vi "ReadStringData.vi"(8 "Error In":errorcluster caption="エラー入力", 10 "データ":T2, 11 "refnum":T1) -> (0 "Error Out":errorcluster caption="エラー出力", 2 "文字列":string, 3 "refnum out":T1 caption="refnum出力")   [LabVIEW 2014]
doc: "iniファイルから文字列データを読み込みます。"
uses:
  <vilib>/Utility/config.llb/NI_LVConfig.lvlib
  <vilib>/Utility/config.llb/Write Key (String).vi
  <vilib>/Utility/config.llb/Read Key (String).vi
  <vilib>/Utility/config.llb/Config Data RefNum.ctl
panel:
  # "■Iniファイルから文字列データを読込む"
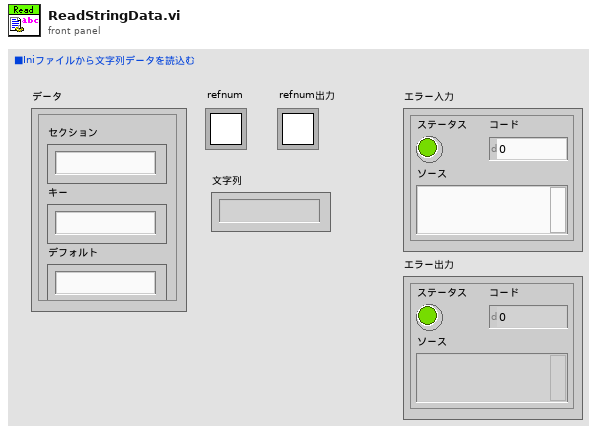
[diagram p1: front panel]
types:
  T1 = typedef "NI_LVConfig.lvlib/Config Data RefNum.ctl" = refnum<k1>
  T2 = cluster{"セクション":string, "キー":string, "デフォルト":string}
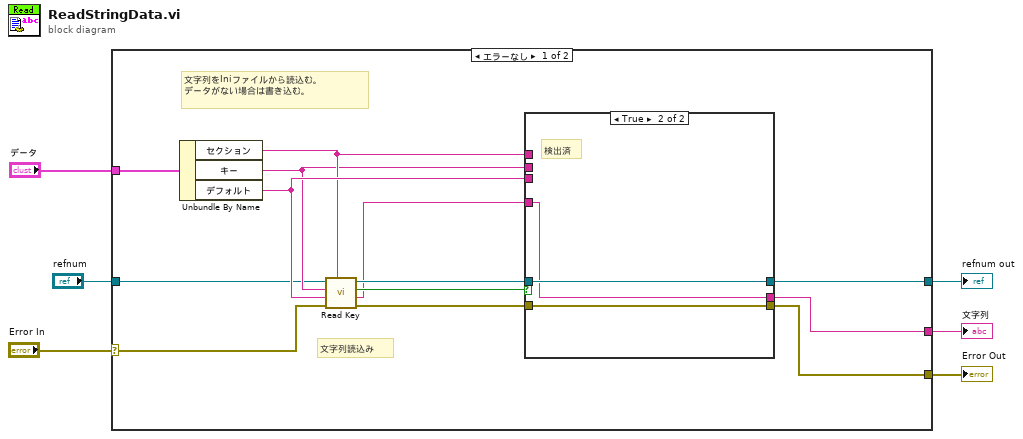
[diagram p0: block diagram]
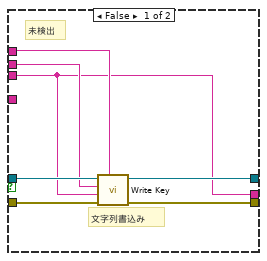
[diagram p2: hidden frame]
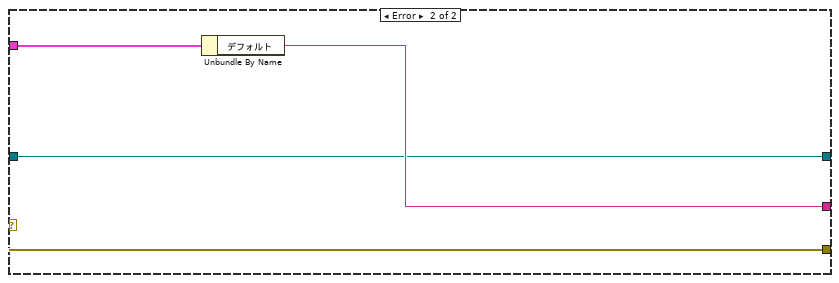
[diagram p3: hidden frame]
diagram:
  n1 = case shown="エラーなし" "Error In" {
    selector: "Error In" -> [w12 w33]
    tunnel: [w13 w33] -> w6
    tunnel: [w11 w31] -> w4
    tunnel: "データ" -> [w10 w32]
    tunnel: [w9 w30] -> w2
    tunnel: "refnum" -> [w8 w30]
    frame No Error {
      # "文字列をIniファイルから読込む。\nデータがない場合は書き込む。"
      # "文字列読込み"
      n2 = Unbundle By Name(w10) -> ("セクション"=w15:string, "キー"=w14:string, "デフォルト"=w16:string)
      n3 = call-poly <vilib>:"Read Key.vi"("section"=w15, "error in (no error)"=w12, "default value"=w16, "key"=w14, "refnum"=w8) -> ("error out"=w17:errorcluster, "value"=w7:string, "found?"=w19:bool, "refnum out"=w18:T1)  [unwired: 3 in]
      n4 = case shown="TRUE" w19 {
        tunnel: w18 -> [w26 w29]
        tunnel: [w25 w29] -> w9
        tunnel: [w20 w27] -> w11
        tunnel: w17 -> [w24 w28]
        tunnel: [w23 w28] -> w13
        tunnel: w16 -> [w20 _]
        tunnel: w15 -> [w22 _]
        tunnel: w14 -> [w21 _]
        tunnel: w7 -> [_ w27]
        frame False {
          # "文字列書込み"
          # "未検出"
          n5 = call-poly <vilib>:"Write Key.vi"("section"=w22, "error in (no error)"=w24, "value"=w20, "key"=w21, "refnum"=w26) -> ("error out"=w23:errorcluster, "refnum out"=w25:T1)  [unwired: 4 in, 1 out]
        }
        frame True {
          # "検出済"
        }
      }
    }
    frame Error {
      n6 = Unbundle By Name(w32) -> ("デフォルト"=w31:string)
    }
  }
  "Error Out" <- w6
  "文字列" <- w4
  "refnum out" <- w2
